vi "Accelerometer.vi"(8 "Accel Range":T2, 11 "Mode":enum8{"Start", "Run", "Finish"}(ring)) -> ()   [LabVIEW 2014]
uses:
  <vilib>/Rock Robotics/WPI/Accelerometer/WPI_AccelerometerRange.ctl
  <vilib>/Rock Robotics/WPI/Accelerometer/InternalAccelerometer/WPI_AccelerometerInternalOpen.vi
  <vilib>/Analysis/NI_AALPro.lvlib
panel:
  out "Z Distance":dbl[](graph)
  out "Y Distance":dbl[](graph)
  out "X Distance":dbl[](graph)
  out "Waveform Chart":T1(graph)
  out "Z Acceleration":dbl
  out "Y Acceleration":dbl
  out "X Acceleration":dbl
  # "Set these inputs before running."
  # "Output information"
  # "This uses the internal accelerometer built into the roboRIO.  No wiring is necessary."
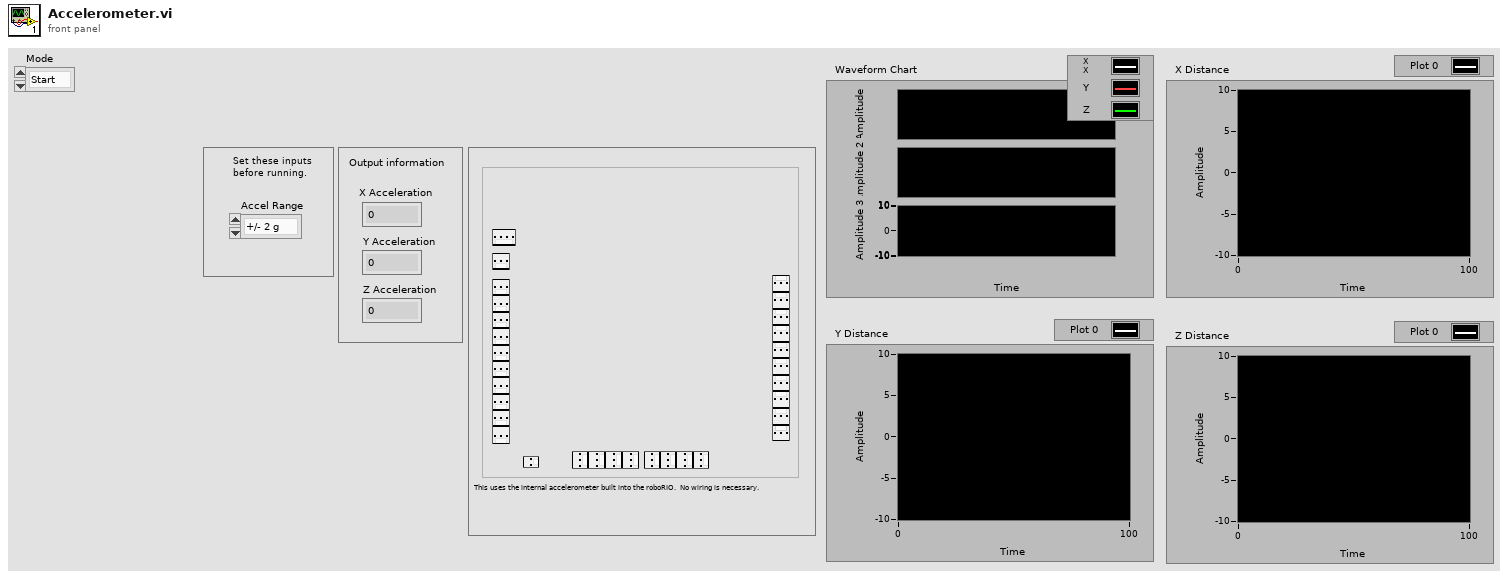
[diagram p1: front panel]
types:
  T1 = cluster{"X-Axis":dbl, "Y-Axis":dbl, "Z-Axis":dbl}
  T2 = typedef "WPI_AccelerometerRange.ctl" = enum16{"+/- 2 g", "+/- 4 g", "+/- 8 g"}
  T3 = typedef "WPI_AccelerometerDevRef.ctl" = cluster{"DevStatus":errorcluster, "Controller":T4, "Scaling":T5, "Analog Channels":T6, "I2C Bus":T8, "SPI Bus":T9, "Accel Range":T10, "ADXL345 Axes":T11, "Handle":i32, "Device Address":u8, "Accel Type":enum16{"Analog", "ADXL345 I2C", "ADXL345 SPI", "Internal"}}
  T4 = typedef "FPGA_TypedefAnalogModule.ctl" = enum16{"Controller 1"}
  T5 = typedef "WPI_AccelerometerScaling.ctl" = cluster{"Gain (VoltsPerG)":dbl, "Center Voltage":dbl}
  T6 = typedef "WPI_AccelerometerAnalogChannels.ctl" = cluster{"X-Axis":T7, "Y-Axis":T7, "Z-Axis":T7}
  T7 = typedef "FPGA_AIChannel.ctl" = enum8{"AI 0", "AI 1", "AI 2", "AI 3", "AI MXP 0", "AI MXP 1", "AI MXP 2", "AI MXP 3", "Invalid"}
  T8 = typedef "i2c_bus.ctl" = enum16{"I2C On-Board", "I2C MXP", "Invalid"}
  T9 = typedef "spi_bus.ctl" = enum16{"SPI On-Board, CS0", "SPI On-Board, CS1", "SPI On-Board, CS2", "SPI On-Board, CS3", "SPI MXP", "Invalid"}
  T10 = typedef "ADXL345 Range.ctl" = u8
  T11 = typedef "WPI_AccelerometerADXL345 Axes.ctl" = cluster{"X-Axis":bool, "Y-Axis":bool, "Z-Axis":bool}
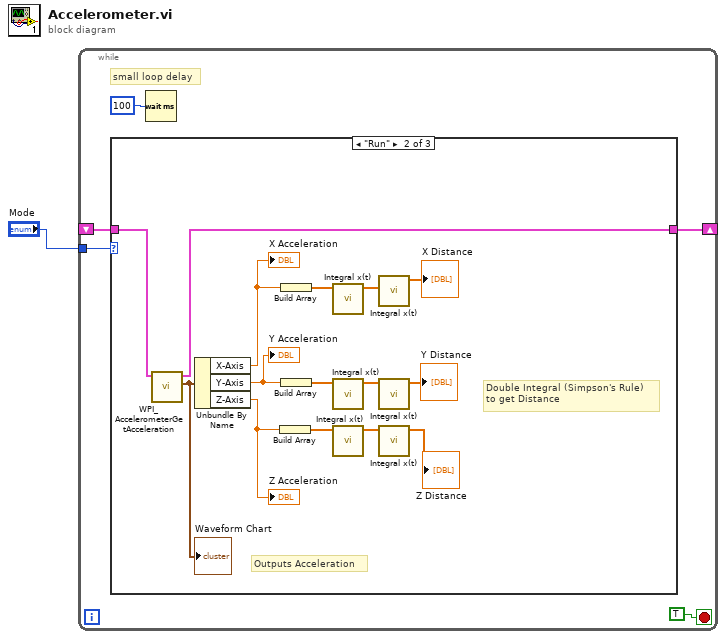
[diagram p0: block diagram]
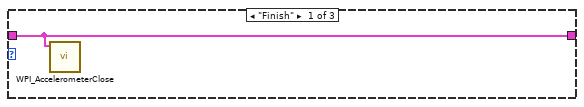
[diagram p2: hidden frame]
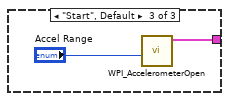
[diagram p3: hidden frame]
diagram:
  n1 = while {
    tunnel: "Mode" -> [w6]
    shift-right: [w4] -> _
    shift-left: _ -> [w3]
    stop <- TRUE stop-if-true
    # "small loop delay"
    n2 = case shown="\"Run\"" w6 {
      tunnel: [w7 w8 w23] -> w4
      tunnel: w3 -> [w7 w22 _]
      frame "Finish" {
        n3 = call <vilib>:"WPI_AccelerometerClose.vi"("AccelerometerDevRef"=w7) -> ()  [unwired: 10 in, 1 out]
      }
      frame "Run" {
        # "Double Integral (Simpson's Rule)\nto get Distance"
        # "Outputs Acceleration"
        n4 = call <vilib>:"WPI_AccelerometerGetAcceleration.vi"("AccelerometerDevRef"=w22) -> ("Accelerations"=w21:T1, "AccelerometerDevRef"=w8:T3)  [unwired: 8 in, 1 out]
        "Waveform Chart" <- w21
        n5 = Unbundle By Name(w21) -> ("X-Axis"=w20:dbl, "Y-Axis"=w17:dbl, "Z-Axis"=w18:dbl)
        "X Acceleration" <- w20
        "Y Acceleration" <- w17
        "Z Acceleration" <- w18
        n6 = Build Array(w18) -> (w15:dbl[])
        n7 = Build Array(w20) -> (w19:dbl[])
        n8 = Build Array(w17) -> (w16:dbl[])
        n9 = call <vilib>:"Integral x(t).vi"("X"=w19) -> ("Integral X"=w13:dbl[])  [unwired: 9 in, 1 out]
        n10 = call <vilib>:"Integral x(t).vi"("X"=w16) -> ("Integral X"=w14:dbl[])  [unwired: 9 in, 1 out]
        n11 = call <vilib>:"Integral x(t).vi"("X"=w15) -> ("Integral X"=w12:dbl[])  [unwired: 9 in, 1 out]
        n12 = call <vilib>:"Integral x(t).vi"("Initial Condition"=w13) -> ("Integral X"=→"X Distance":dbl[])  [unwired: 9 in, 1 out]
        n13 = call <vilib>:"Integral x(t).vi"("X"=w14) -> ("Integral X"=→"Y Distance":dbl[])  [unwired: 9 in, 1 out]
        n14 = call <vilib>:"Integral x(t).vi"("X"=w12) -> ("Integral X"=→"Z Distance":dbl[])  [unwired: 9 in, 1 out]
      }
      frame "Start", Default {
        n15 = call-poly <vilib>:"WPI_AccelerometerOpen.vi"("Accel Range"="Accel Range") -> ("AccelerometerDevRef"=w23:T3)  [unwired: 9 in, 1 out]
      }
    }
    n16 = Wait (ms)(milliseconds to wait=u32 100) -> ()  [unwired: 1 out]
  }
